vi "LUT.CreateEntry.vi"(7 "Type":T1=enum."Input/Read", 8 "error in (no error)":errorcluster, 10 "Name":string, 11 "LUT":variant) -> (0 "error out":errorcluster, 3 "LUT":variant)   [LabVIEW 2015, in "Data Access System Explorer.lvlib"]
uses:
  Data Access System Explorer.lvlib
  Types/VS Channel Group Type.ctl
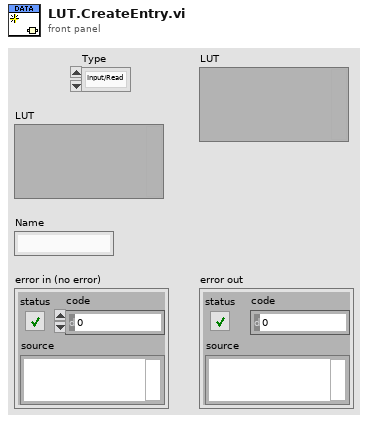
[diagram p1: front panel]
types:
  T1 = typedef "Data Access System Explorer.lvlib/VS Channel Group Type.ctl" = enum16{"Output/Write", "Input/Read", "Input/ReadWrite"}
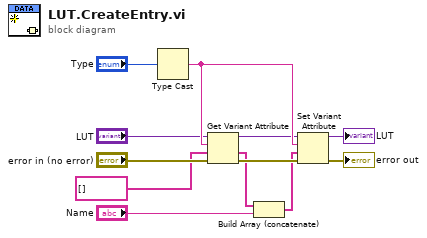
[diagram p0: block diagram]
diagram:
  n1 = Type Cast(x="Type") -> (*(type *) &x=w5:string)  [unwired: 1 in]
  n2 = Get Variant Attribute(Variant="LUT", name=w5, default value (empty Variant)=string[] [], error in="error in (no error)") -> (duplicate Variant=w3:variant, value=w7:string[], error out=w10:errorcluster)  [unwired: 1 out]
  n3 = Build Array (concatenate)(w7, "Name") -> (w8:string[])
  n4 = Set Variant Attribute(Variant=w3, name=w5, value=w8, error in=w10) -> (Variant out=→"LUT":variant, error out=→"error out":errorcluster)  [unwired: 1 out]
